vi "Read Channels.vi"(8 "error in":errorcluster, 11 "execution unit in":refnum<class "Execution Unit.lvclass">) -> (0 "error out":errorcluster, 2 "channels":u8[](array[numeric]), 3 "execution unit out":refnum<class "Execution Unit.lvclass">)   [LabVIEW 2020, in "AIM ARINC 429 Engine.lvlib" / "Implementation.lvlib" / "Execution Unit.lvclass"]
uses:
  Execution Unit.lvclass
  Execution Unit.lvclass/Execution Unit.ctl
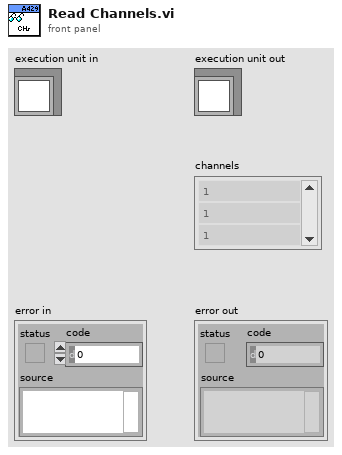
[diagram p1: front panel]
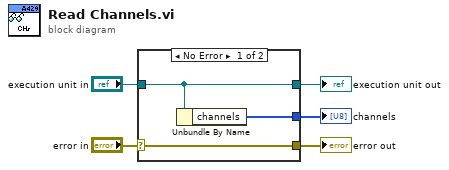
[diagram p0: block diagram]
diagram:
  n1 = case shown="No Error" "error in" {
    selector: "error in" -> [w8 w9]
    tunnel: [w8 w9] -> w4
    tunnel: [w7 w10] -> w2
    tunnel: "execution unit in" -> [w7 w10]
    tunnel: [w6 _] -> w1
    frame No Error {
      n2 = Unbundle By Name(w7) -> ("channels"=w6:u8[])
    }
    frame Error {
    }
  }
  "error out" <- w4
  "execution unit out" <- w2
  "channels" <- w1
